vi "Manual_batch_DCIMG_metadataread_single_color_only.vi"() -> ()   [LabVIEW 2016]
panel:
  out "size(s)":i32
  out "inter-volume time":i32[](array[numeric])
  out "metadata strings":string[](array[string])
  out "current file number":i32
  in  "Select dataset folder (the folder that houses the SPIMA and SPIMB folders)":path
  out "error IO":errorcluster
  # "This program will read the metadata written into DCIMG files \nand display the time interval between the consecutive timeframes.\nThis information is important for calculating the durations and \nspeed of tracks during analysis."
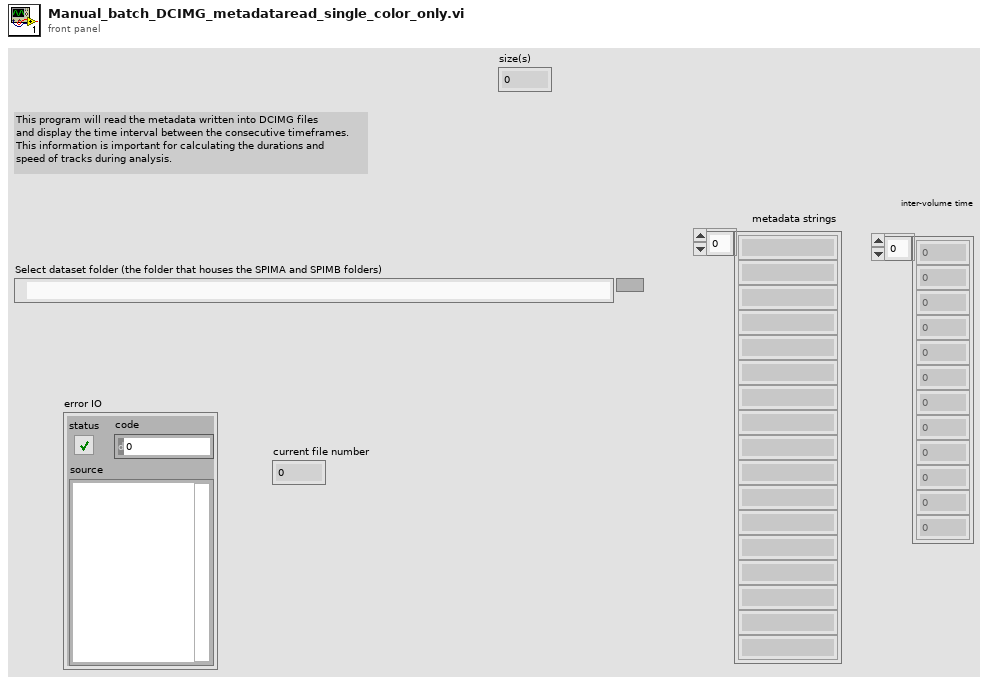
[diagram p1: front panel]
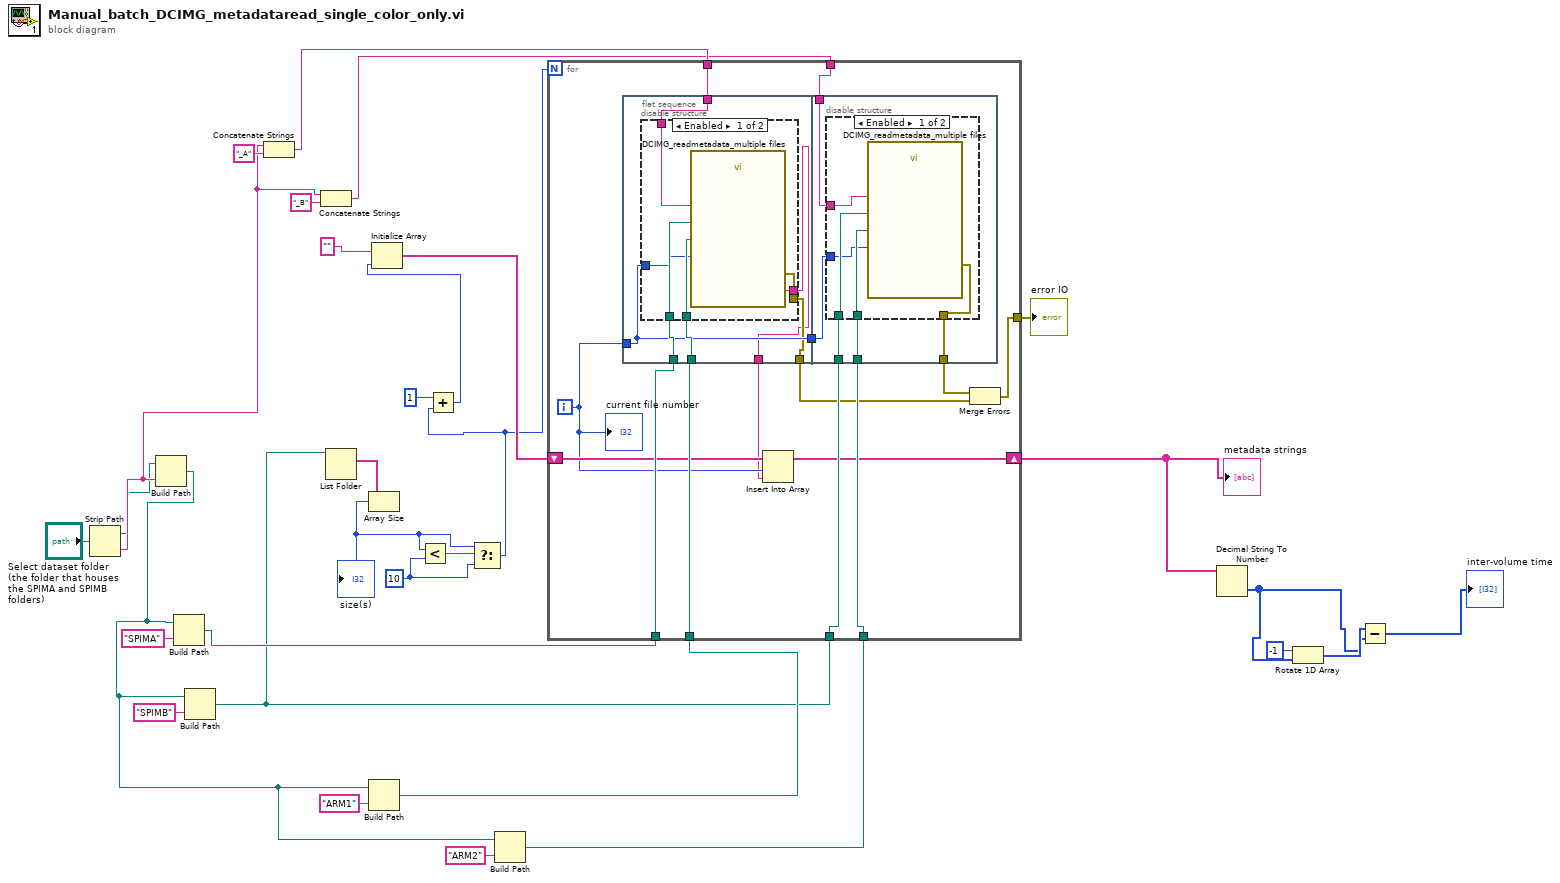
[diagram p0: block diagram]
diagram:
  w2 = 10
  n1 = Strip Path(path="Select dataset folder (the folder that houses the SPIMA and SPIMB folders)") -> (stripped path=w15:path, name=w16:string)
  n2 = Build Path(base path=w15, name or relative path=w16) -> (appended path=w21:path)
  n3 = Build Path(base path=w21, name or relative path="SPIMA") -> (appended path=w18:path)
  n4 = Build Path(base path=w21, name or relative path="SPIMB") -> (appended path=w14:path)
  n5 = Concatenate Strings(w16, "_A" ("string")) -> (w26:string)
  n6 = Concatenate Strings(w16, "_B" ("string")) -> (w24:string)
  n7 = List Folder(path=w14) -> (filenames=w31:string[])  [unwired: 3 in, 3 out]
  n8 = Array Size(array=w31) -> (size(s)=w3:i32)
  "size(s)" <- w3
  n9 = Build Path(base path=w21, name or relative path="ARM1") -> (appended path=w22:path)
  n10 = Less?(x=w3, y=w2) -> (x < y?=w4:bool)
  n11 = Select(t=w3, s=w4, f=w2) -> (s? t:f=w1:i32)
  n12 = Add(x=1, y=w1) -> (x+y=w12:i32)
  n13 = Initialize Array("", w12) -> (w10:string[])
  n14 = Build Path(base path=w21, name or relative path="ARM2") -> (appended path=w19:path)
  n15 = for {
    N: w1 -> [_]
    tunnel: w18 -> [w45]
    tunnel: w14 -> [w44]
    tunnel: [w38] -> w30
    tunnel: w22 -> [w43]
    tunnel: w19 -> [w42]
    tunnel: w26 -> [w37]
    tunnel: w24 -> [w36]
    shift-right: [w32] -> w9
    shift-left: w10 -> [w35]
    i -> [w34]
    n16 = flat-sequence {
      tunnel: w45 -> [w51]
      tunnel: w34 -> [w49]
      tunnel: w43 -> [w50]
      tunnel: [w49] -> w41
      tunnel: [w48] -> w39
      tunnel: w37 -> [w47]
      tunnel: [w46] -> w33
      tunnel: w44 -> [w62]
      tunnel: w42 -> [w61]
      tunnel: w41 -> [w60]
      tunnel: [w59] -> w40
      tunnel: w36 -> [w58]
      frame #0 {
        n17 = disable-structure shown="Enabled" {
          disable-tunnel: w51 -> [w57 _]
          disable-tunnel: w50 -> [w56 _]
          disable-tunnel: w49 -> [w55 _]
          disable-tunnel: [w54 _] -> w48
          disable-tunnel: w47 -> [w53 _]
          disable-tunnel: [w52 _] -> w46
          frame Enabled {
            n18 = call "DCIMG_readmetadata_multiple files.vi"("Volume number"=w55, "Input File Path"=w57, "Input File Name"=w53, "Output Path"=w56) -> ("Metadata"=w52:string, "Error Out"=w54:errorcluster)  [unwired: 9 in, 1 out]
          }
          frame Disabled {
          }
        }
      }
      frame #1 {
        n19 = disable-structure shown="Enabled" {
          disable-tunnel: w62 -> [w67 _]
          disable-tunnel: w61 -> [w66 _]
          disable-tunnel: w60 -> [w65 _]
          disable-tunnel: [w64 _] -> w59
          disable-tunnel: w58 -> [w63 _]
          frame Enabled {
            n20 = call "DCIMG_readmetadata_multiple files.vi"("Volume number"=w65, "Input File Path"=w67, "Input File Name"=w63, "Output Path"=w66) -> ("Error Out"=w64:errorcluster)  [unwired: 9 in, 2 out]
          }
          frame Disabled {
          }
        }
      }
    }
    n21 = Insert Into Array(array=w35, index=w34, new element=w33) -> (w32:string[])
    n22 = Merge Errors(w40, w39) -> (w38:errorcluster)
    "current file number" <- w34
  }
  "error IO" <- w30
  "metadata strings" <- w9
  n23 = Decimal String To Number(string=w9) -> (number=w5:i32[])  [unwired: 2 in, 1 out]
  n24 = Rotate 1D Array(1:w5, 2:-1 ("n")) -> (0:w6:i32[])
  n25 = Subtract(x=w6, y=w5) -> (x-y=→"inter-volume time":i32[])
